vi "WLAN - TV - RW - UTIL - StringClusterToDataType(Meas).vi"(7 "TV Paramaters(String)":T2) -> (8 "TV Parameters(DataType)":T1 {"Tx_Chan" format="%.0x"; "Standard" items=["80211A/G/J/P OFDM", "80211B/G DSSS", "80211G DSSSOFDM", "80211N MIMOOFDM", "80211AC MIMOOFDM"]; "OFDM Data Rate (Mbps)" items=["6", "9", "12", "18", "24", "36", "48", "54"]; "80211n PLCP Frame Format" items=["Mixed Format", "Greenfield Format"]; "FEC Coding Type" items=["BCC", "LDPC"]; "DSSS Data Rate (Mbps)" items=["1", "2", "5.5 CCK", "5.5 PBCC", "11 CCK", "11 PBCC", "22", "33"]})   [LabVIEW 2011]
uses:
  Includes/WLAN - TV - RW - INC - TV_Parameters.ctl
  Includes/WLAN - TV - RW - INC - TV_DataType_Cluster.ctl
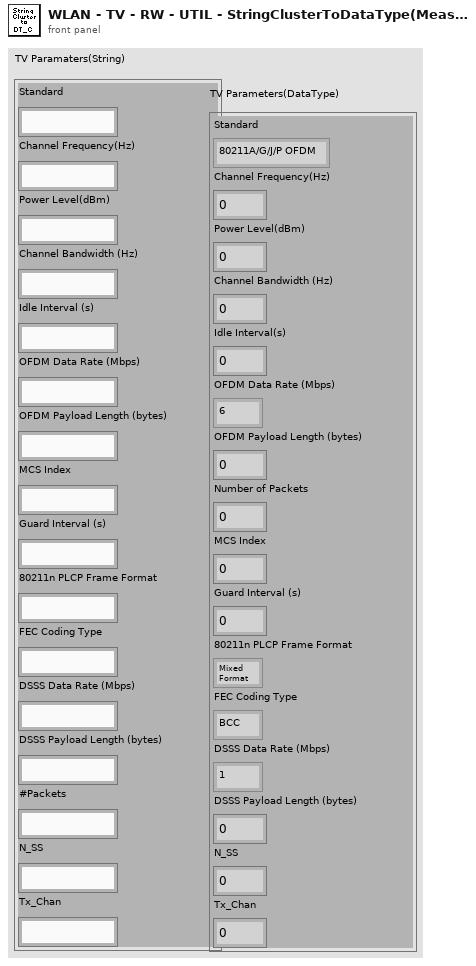
[diagram p1: front panel]
types:
  T1 = typedef "WLAN - TV - RW - INC - TV_DataType_Cluster.ctl" = cluster{"Standard":i32, "Channel Frequency(Hz)":dbl, "Power Level(dBm)":dbl, "Channel Bandwidth (Hz)":dbl, "Idle Interval(s)":dbl, "OFDM Data Rate (Mbps)":i32, "OFDM Payload Length (bytes)":i32, "Number of Packets":i32, "MCS Index":i32, "Guard Interval (s)":dbl, "80211n PLCP Frame Format":i32, "FEC Coding Type":i32, "DSSS Data Rate (Mbps)":i32, "DSSS Payload Length (bytes)":i32, "N_SS":i32, "Tx_Chan":u32}
  T2 = typedef "WLAN - TV - RW - INC - TV_Parameters.ctl" = cluster{"Standard ":string, "Channel Frequency(Hz)":string, "Power Level(dBm)":string, "Channel Bandwidth (Hz)":string, "Idle Interval (s)":string, "OFDM Data Rate (Mbps)":string, "OFDM Payload Length (bytes)":string, "MCS Index":string, "Guard Interval (s)":string, "80211n PLCP Frame Format":string, "FEC Coding Type":string, "DSSS Data Rate (Mbps)":string, "DSSS Payload Length (bytes)":string, "#Packets":string, "N_SS":string, "Tx_Chan":string}
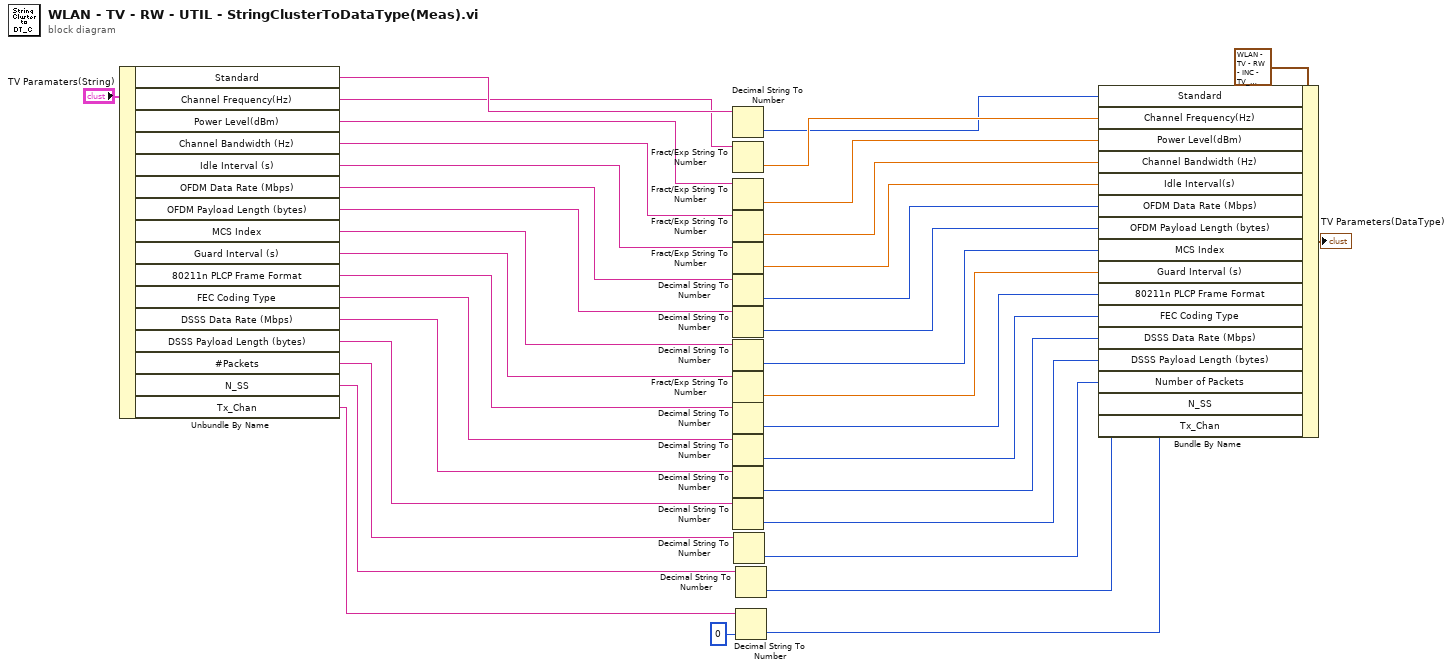
[diagram p0: block diagram]
diagram:
  n1 = Unbundle By Name("TV Paramaters(String)") -> ("Standard"=w34:string, "Channel Frequency(Hz)"=w33:string, "Power Level(dBm)"=w32:string, "Channel Bandwidth (Hz)"=w31:string, "Idle Interval (s)"=w30:string, "OFDM Data Rate (Mbps)"=w29:string, "OFDM Payload Length (bytes)"=w28:string, "MCS Index"=w27:string, "Guard Interval (s)"=w26:string, "80211n PLCP Frame Format"=w25:string, "FEC Coding Type"=w24:string, "DSSS Data Rate (Mbps)"=w23:string, "DSSS Payload Length (bytes)"=w22:string, "#Packets"=w10:string, "N_SS"=w5:string, "Tx_Chan"=w3:string)
  n2 = Decimal String To Number(string=w34) -> (number=w12:i32)  [unwired: 2 in, 1 out]
  n3 = Fract/Exp String To Number(string=w33) -> (number=w13:dbl)  [unwired: 3 in, 1 out]
  n4 = Fract/Exp String To Number(string=w32) -> (number=w8:dbl)  [unwired: 3 in, 1 out]
  n5 = Fract/Exp String To Number(string=w31) -> (number=w14:dbl)  [unwired: 3 in, 1 out]
  n6 = Fract/Exp String To Number(string=w30) -> (number=w15:dbl)  [unwired: 3 in, 1 out]
  n7 = Decimal String To Number(string=w29) -> (number=w16:i32)  [unwired: 2 in, 1 out]
  n8 = Decimal String To Number(string=w28) -> (number=w17:i32)  [unwired: 2 in, 1 out]
  n9 = Decimal String To Number(string=w27) -> (number=w18:i32)  [unwired: 2 in, 1 out]
  n10 = Fract/Exp String To Number(string=w26) -> (number=w6:dbl)  [unwired: 3 in, 1 out]
  n11 = Decimal String To Number(string=w25) -> (number=w19:i32)  [unwired: 2 in, 1 out]
  n12 = Decimal String To Number(string=w24) -> (number=w20:i32)  [unwired: 2 in, 1 out]
  n13 = Decimal String To Number(string=w23) -> (number=w21:i32)  [unwired: 2 in, 1 out]
  n14 = Decimal String To Number(string=w22) -> (number=w11:i32)  [unwired: 2 in, 1 out]
  n15 = Decimal String To Number(string=w10) -> (number=w7:i32)  [unwired: 2 in, 1 out]
  n16 = Decimal String To Number(string=w5) -> (number=w4:i32)  [unwired: 2 in, 1 out]
  n17 = Decimal String To Number(string=w3, default (0L)=u32 0 ("default (0 I32)")) -> (number=w1:u32)  [unwired: 1 in, 1 out]
  n18 = Bundle By Name(cluster=T1 {"Standard"=0, "Channel Frequency(Hz)"=0.0, "Power Level(dBm)"=0.0, "Channel Bandwidth (Hz)"=0.0, "Idle Interval(s)"=0.0, "OFDM Data Rate (Mbps)"=0, "OFDM Payload Length (bytes)"=0, "Number of Packets"=0, "MCS Index"=0, "Guard Interval (s)"=0.0, "80211n PLCP Frame Format"=0, "FEC Coding Type"=0, "DSSS Data Rate (Mbps)"=0, "DSSS Payload Length (bytes)"=0, "N_SS"=0, "Tx_Chan"=0} ("TV Parameters(DataType)"), "Standard"=w12, "Channel Frequency(Hz)"=w13, "Power Level(dBm)"=w8, "Channel Bandwidth (Hz)"=w14, "Idle Interval(s)"=w15, "OFDM Data Rate (Mbps)"=w16, "OFDM Payload Length (bytes)"=w17, "MCS Index"=w18, "Guard Interval (s)"=w6, "80211n PLCP Frame Format"=w19, "FEC Coding Type"=w20, "DSSS Data Rate (Mbps)"=w21, "DSSS Payload Length (bytes)"=w11, "Number of Packets"=w7, "N_SS"=w4, "Tx_Chan"=w1) -> (→"TV Parameters(DataType)":T1)
